vi "Setup DMM Channels.vi"(0 "TSM Context":T1, 11 "error in":errorcluster) -> (15 "error out":errorcluster)   [LabVIEW 2019]
uses:
  <vilib>/NI_TestStand_SemiconductorModule/NI_TestStand_Semiconductor_Module.lvlibp/PinMap/General/SemiconductorModuleContext.ctl
  <instrlib>/niDMM/nidmm.llb/niDMM Function.ctl
  <instrlib>/niDMM/nidmm.llb/niDMM Resolution in Digits.ctl
  <vilib>/NI_TestStand_SemiconductorModule/NI_TestStand_Semiconductor_Module.lvlibp
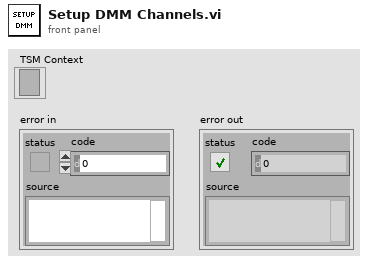
[diagram p1: front panel]
types:
  T1 = typedef "NI_TestStand_Semiconductor_Module.lvlibp/SemiconductorModuleContext.ctl" = refnum<k7>
  T2 = typedef "niDMM Resolution in Digits.ctl" = dbl
  T3 = typedef "niDMM Function.ctl" = enum16{"DC Volts", "AC Volts", "DC Current", "AC Current", "2-wire Resistance", "4-wire Resistance", "Diode", "Frequency", "Period", "AC Volts DC Coupled", "Capacitance", "Inductance", "Temperature"}
  T4 = typedef "TSM DMM.ctl" = cluster{"Pin Query Context":refnum<class "MultiplePinMultipleSessionQueryContext.lvclass">, "Sessions":refnum<k15>[]}
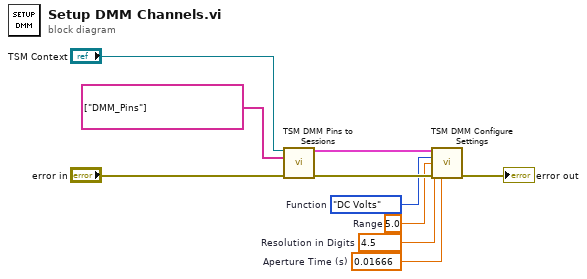
[diagram p0: block diagram]
diagram:
  w1 = 0.01666  # Aperture Time (s)
  w2 = T2 4.5 items=["3 1/2"=3.5, "4 1/2"=4.5, "5 1/2"=5.5, "6 1/2"=6.5, "7 1/2"=7.5]  # Resolution in Digits
  w3 = 5.0  # Range
  w4 = niDMM_Function."DC Volts"  # Function
  n1 = call "TSM DMM Pins to Sessions.vi"("TSM Context"="TSM Context", "Pins"=tag[] ["DMM_Pins"], "error in"="error in") -> ("DMM TSM Out"=w7:T4, "error out"=w6:errorcluster)  [unwired: 11 in]
  n2 = call "TSM DMM Configure Settings.vi"("DMM TSM In"=w7, "Function"=w4, "Range"=w3, "Resolution in Digits"=w2, "error in"=w6, "Aperture Time (s)"=w1) -> ("error out"=→"error out":errorcluster)  [unwired: 8 in, 1 out]
